vi "Configure Integration Current.vi"(5 "Element (0: ALL)":i32(ring) items=["All", "1", "2", "3", "4", "5", "6"], 8 "error in (no error)":errorcluster, 10 "Current Mode (2: dc)":i32(ring)=2 items=["rms", "mean", "dc", "r-mean", "ac"], 11 "VISA resource name":refnum<visa-resource-name>) -> (0 "error out":errorcluster, 3 "VISA resource name out":refnum<visa-resource-name>)   [LabVIEW 2021, in "Yokogawa WT1800 Series.lvlib"]
doc: "Configures the current mode for current integration features."
uses:
  <instrlib>/Yokogawa WT1800 Series/Yokogawa WT1800 Series.lvlib
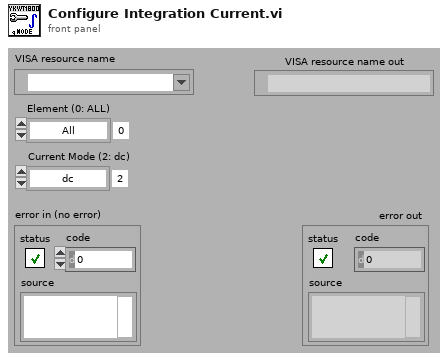
[diagram p1: front panel]
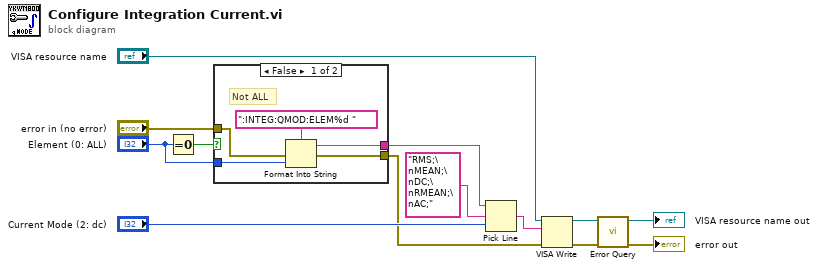
[diagram p0: block diagram]
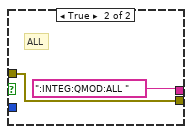
[diagram p2: hidden frame]
diagram:
  n1 = Equal To 0?(x="Element (0: ALL)") -> (x = 0?=w8:bool)
  n2 = case shown="False" w8 {
    tunnel: "error in (no error)" -> [w17 w20]
    tunnel: [w16 w20] -> w2
    tunnel: [w15 ":INTEG:QMOD:ALL "] -> w1
    tunnel: "Element (0: ALL)" -> [w14 _]
    frame False {
      # "Not ALL"
      n3 = Format Into String ("文字列にフォーマット")(format string=":INTEG:QMOD:ELEM%d " ("形式文字列"), error in=w17, w14) -> (resulting string=w15:string, error out=w16:errorcluster)  [unwired: 1 in]
    }
    frame True {
      # "ALL"
    }
  }
  n4 = Pick Line ("ライン選択")(string ("")=w1, multi-line string="RMS;\nMEAN;\nDC;\nRMEAN;\nAC;" ("複数行文字列"), line index="Current Mode (2: dc)") -> (output string=w3:string)
  n5 = VISA Write ("VISA書き込み")(VISA resource name="VISA resource name", write buffer=w3, error in (no error)=w2) -> (VISA resource name out=w13:refnum<visa-resource-name>, error out=w12:errorcluster)  [unwired: 1 out]
  n6 = call <instrlib>:"Error Query.vi"("error in (no error)"=w12, "VISA resource name"=w13) -> ("error out"=→"error out":errorcluster, "VISA resource name out"=→"VISA resource name out":refnum<visa-resource-name>)  [unwired: 6 in, 2 out]
